vi "ARRAY.vi"() -> ()   [LabVIEW 2018]
panel:
  out "output array":dbl[][](array[numeric])
  out "sorted array":dbl[](array[numeric])
  in  "row to sort":dbl
  out "Array":dbl[][](array[numeric])
  in  "column":dbl
  in  "rows":dbl
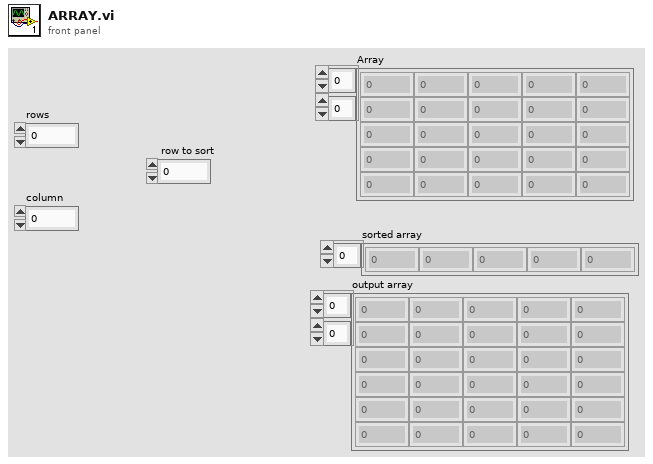
[diagram p1: front panel]
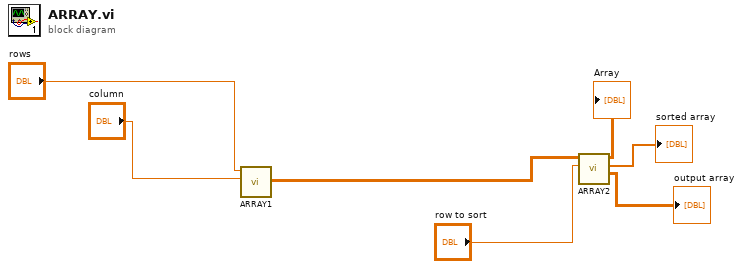
[diagram p0: block diagram]
diagram:
  n1 = call "ARRAY1.vi"("Numeric 2"="column", "Numeric"="rows") -> ("Array 2"=w5:dbl[][])  [unwired: 9 in]
  n2 = call "ARRAY2.vi"("row to sort"="row to sort", "Array in"=w5) -> ("output array"=→"output array":dbl[][], "sorted array"=→"sorted array":dbl[], "Array out"=→"Array":dbl[][])  [unwired: 7 in]
